vi "Write Source.vi"(8 "error in (no error)":errorcluster, 10 "Source":string, 11 "Event in":refnum<class "Event.lvclass">) -> (0 "error out":errorcluster, 3 "Event out":refnum<class "Event.lvclass">)   [LabVIEW 2013, in "Event.lvclass"]
uses:
  Event.lvclass
  Event.lvclass/Event.ctl
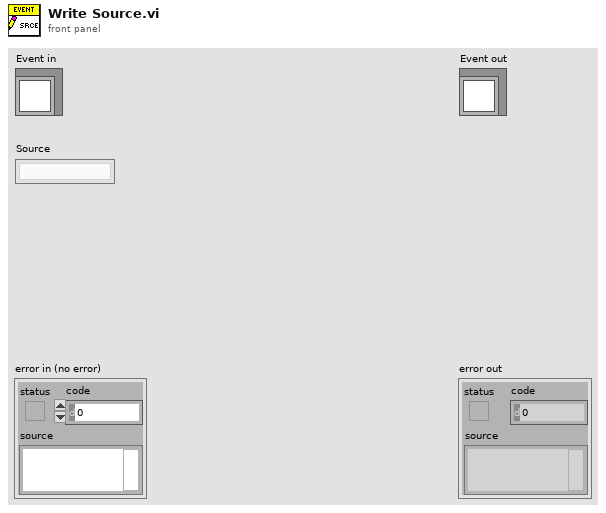
[diagram p1: front panel]
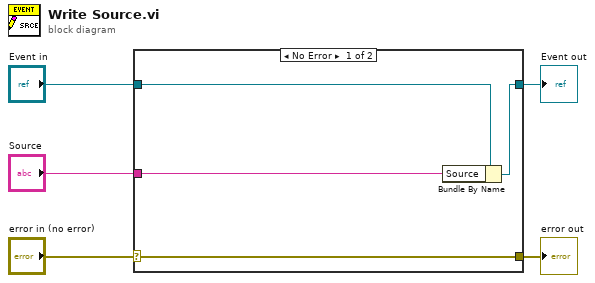
[diagram p0: block diagram]
diagram:
  n1 = case shown="No Error" "error in (no error)" {
    selector: "error in (no error)" -> [w9 w10]
    tunnel: [w9 w10] -> w4
    tunnel: [w7 w11] -> w2
    tunnel: "Event in" -> [w8 w11]
    tunnel: "Source" -> [w6 _]
    frame No Error {
      n2 = Bundle By Name(cluster=w8, "Source"=w6) -> (w7:refnum<class "Event.lvclass">)
    }
    frame Error {
    }
  }
  "error out" <- w4
  "Event out" <- w2
